vi "Coord window-Normalise main screen coord for display.vi"(9 "Motor coordinates":cluster{"X":sgl, "Y":sgl, "Z":sgl}, 11 "Picture map ref in":refnum<vi>) -> (1 "Normalised top level screen coordinates (for display)":cluster{"x":i16, "y":i16}, 3 "Picture map ref":refnum<vi>)   [LabVIEW 2020]
uses:
  Globals/Coord window-Globals.vi
  <vilib>/gmath/NI_Gmath.lvlib
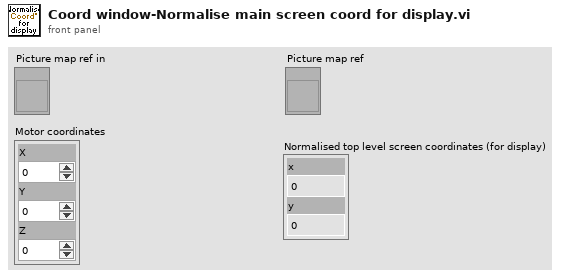
[diagram p1: front panel]
types:
  T1 = typedef "LVBoundsTypeDef.ctl" = cluster{"Width":u32, "Height":u32}
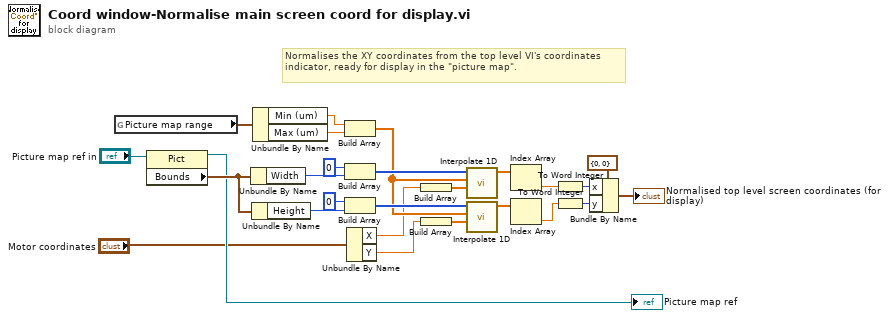
[diagram p0: block diagram]
diagram:
  # "Normalises the XY coordinates from the top level VI's coordinates indicator, ready for display in the \"picture map\"."
  n1 = global read "Coord window-Globals.vi" "Picture map range"() -> (w20:cluster{"Min (um)":dbl, "Max (um)":dbl})
  n2 = property on="Property Node" class="Pict"(reference="Picture map ref in") -> (reference out=→"Picture map ref":refnum<vi>, "Bounds"=w4:T1)  [unwired: 1 in, 1 out]
  n3 = Unbundle By Name(w4) -> ("Width"=w21:u32)
  n4 = Unbundle By Name(w4) -> ("Height"=w24:u32)
  n5 = Unbundle By Name(w20) -> ("Min (um)"=w19:dbl, "Max (um)"=w18:dbl)
  n6 = Build Array(w19, w18) -> (w17:dbl[])
  n7 = Build Array(u32 0 ("element"), w21) -> (w25:u32[])
  n8 = Build Array(u32 0 ("element"), w24) -> (w26:u32[])
  n9 = Unbundle By Name("Motor coordinates") -> ("X"=w7:sgl, "Y"=w6:sgl)
  n10 = Build Array(w7) -> (w16:sgl[])
  n11 = Build Array(w6) -> (w11:sgl[])
  n12 = call <vilib>:"Interpolate 1D.vi"("xi"=w16, "X"=w17, "Y"=w25) -> ("yi"=w15:dbl[])  [unwired: 6 in, 2 out]
  n13 = call <vilib>:"Interpolate 1D.vi"("xi"=w11, "X"=w17, "Y"=w26) -> ("yi"=w12:dbl[])  [unwired: 6 in, 2 out]
  n14 = Index Array(array=w15) -> (element=w13:dbl)  [unwired: 1 in]
  n15 = Index Array(array=w12) -> (element=w10:dbl)  [unwired: 1 in]
  n16 = To Word Integer(number=w13) -> (16bit integer=w9:i16)
  n17 = To Word Integer(number=w10) -> (16bit integer=w8:i16)
  n18 = Bundle By Name(cluster=cluster{"x":i16, "y":i16} {"x"=0, "y"=0} ("point(x,y)"), "x"=w9, "y"=w8) -> (→"Normalised top level screen coordinates (for display)":cluster{"x":i16, "y":i16})
